vi "BuildFRF.vi"(8 "Method":enum16{"Sqrt(H1H2)", "H1", "H2"}(ring), 9 "Settings":T1={"Name of test"="ScratchPad", "Date"=timestamp(0 s since 1904-01-01), "Location"="Home", "Template"="ScratchPad", "Soundcard"="OCTA-CAPTURE", "resolution"=32, "Sampling rate"=48000, "Ch1 Gain "=25.0, "Ch2 Gain"=10.0, "Sample time (s)"=0.3, "Pre-trigger (s)"=0.001, "Hammer Threshold"=10.0, "Positions"=12, "Taps/Position"=5, "Set Names"="H,V", "Freq resolution"=1.0, "Hammer cutoff"=0.025, "Mic cutoff"=0.25, "Double bounce "=10.0, "Hammer Cal"=0.022, "dB Offset"=0.0, "Accel Cal"=10.0, "Vibrometer Cal"=1.0, "Mic Cal"=1.0, "Output"=2, "Voltage Cal"=1.0, "Vibrometer Port"="ASRL27::INSTR", "Range"=4, "High Pass"=2, "Bandwidth"=4, "X Range"=[], "Y Range"=[], "dB Spread"=0.0, "Trigger"=0, "Ch_1"=25, "Ch_2"=25, "flip?"=FALSE, "60Hz"=FALSE, "Time offset"=0.0, "Piezo Cal"=1.0, "Default Notes"=""} {"Ch_2" min=1 step=1; "Ch_1" min=1 max=100 step=1; "Trigger" items=["Hammer (force)", "Self-tap", "Spacebar"]; "Bandwidth" items=["1 kHz"=1, "5 kHz"=5, "10 kHz"=10, "25 kHz"=25, "50 kHz"=50, "100 kHz"=100]; "High Pass" items=["Off", "13 Hz", "104 Hz"]; "Range" items=["10 mm/s"=1, "20 mm/s"=2, "50 mm/s"=5, "100 mm/s"=10, "200 mm/s"=20, "500 mm/s"=50, "1 m/s"=100, "2 m/s"=200]; "Output" items=["Accelerometer", "Speed (from acceleration)", "Microphone", "Vibrometer", "Piezo"]; "Voltage Cal" format="%#_13g"; "Ch2 Gain" format="%#_13g"; "Ch1 Gain" format="%#_13g"; "Double bounce" min=0.0; "Mic cutoff" min=0.0 format="%#_4g"; "Hammer cutoff" min=0.0 format="%#_4g"; "Freq resolution" min=0.0; "Pre-trigger (s)" format="%#_13g"; "Date" format="%<%H:%M\n%d/%m/%y>T"; "resolution" items=["16 bit"=16, "24 bit"=24, "32 bit"=32]; "Sampling rate" items=["22050 samp/s"=22050, "44100 samp/s"=44100, "48000 samp/s"=48000]}, 10 "View":u16(ring) items=["Raw", "Volts", "Units (Pa, N, mm/s etc)"], 11 "Data In":waveform(dbl)[](array[waveform])=[{"t0"=timestamp(3613749982.386897 s since 1904-01-01), "dt"=2.0833333333333333e-05, "Y"=array[14400 elements]}, {"t0"=timestamp(3613749982.386897 s since 1904-01-01), "dt"=2.0833333333333333e-05, "Y"=array[14400 elements]}]) -> (0 "Average FRF":cluster{dbl, "df":dbl, dbl[]}[](graph)=[{1.0, "df"=1.0, array[24000 elements]}, {1.0, "df"=1.0, array[24000 elements]}], 1 "Microphone":cluster{dbl, "dt":dbl, "Y":dbl[]}[](graph)=[{0.0, "dt"=2.0833333333333333e-05, "Y"=array[14400 elements]}], 2 "Hammer":cluster{dbl, "dt":dbl, "Y":dbl[]}[](graph), 3 "Complex FRF":cluster{"t0":dbl, "dt":dbl, "Y":cdb[]}={"t0"=1.0, "dt"=1.0, "Y"=array[24000 elements]}, 4 "Microphone Spectra":cluster{"x0":dbl, "df":dbl, dbl[]}[](graph)=[{"x0"=1.0, "df"=1.0, array[24000 elements]}], 5 "Hammer Spectra":cluster{dbl, "df":dbl, "FFT {X}":dbl[]}[](graph)=[{1.0, "df"=1.0, "FFT {X}"=array[24000 elements]}])   [LabVIEW 2022 SP3]
uses:
  PreferencesControl.ctl
  Mic/Mic_Global.vi
panel:
  # "Always empty for TapTones because there is no hammer"
  # "Hz"
  # "dB"
  # "dB"
  # "sec"
  # "sec"
  # "mV/Pa"
  # "mV/m/s2"
  # "mV/mm/s"
  # "V/N"
  # "sec"
  # "sec"
  # "mV/N"
  # "a.u."
  # "a.u."
  # "sec"
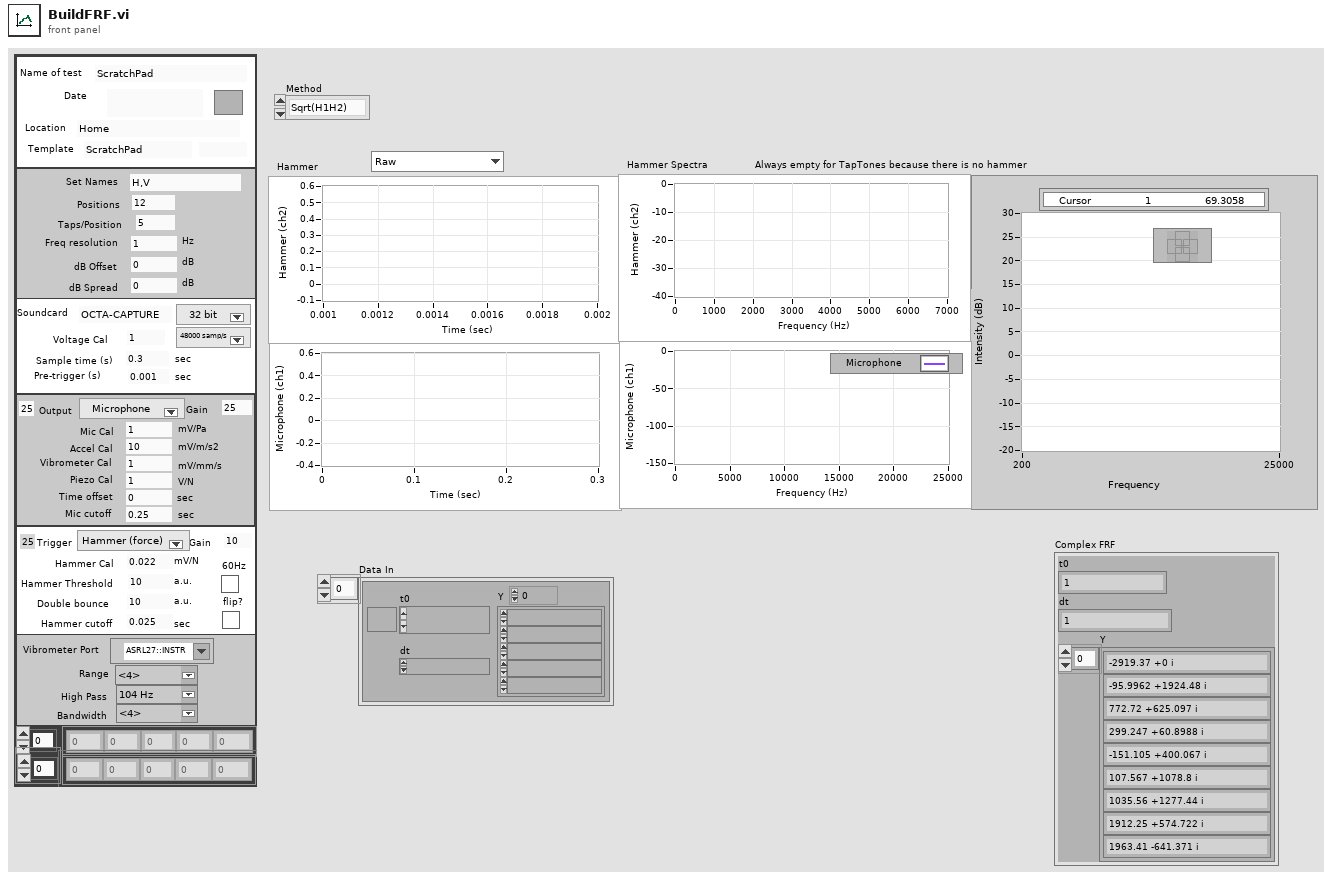
[diagram p1: front panel]
types:
  T1 = typedef "PreferencesControl.ctl" = cluster{"Name of test":string, "Date":timestamp, "Location":string, "Template":string, "Soundcard":string, "resolution":u16, "Sampling rate":u16, "Ch1 Gain ":dbl, "Ch2 Gain":dbl, "Sample time (s)":dbl, "Pre-trigger (s)":dbl, "Hammer Threshold":dbl, "Positions":i16, "Taps/Position":i16, "Set Names":string, "Freq resolution":dbl, "Hammer cutoff":dbl, "Mic cutoff":dbl, "Double bounce ":dbl, "Hammer Cal":dbl, "dB Offset":dbl, "Accel Cal":dbl, "Vibrometer Cal":dbl, "Mic Cal":dbl, "Output":u16, "Voltage Cal":dbl, "Vibrometer Port":refnum<visa-resource-name>, "Range":u16, "High Pass":u16, "Bandwidth":u16, "X Range":cluster{"Minimum":dbl, "Maximum":dbl, "Increment":dbl, "Minor Increment":dbl, "Start":dbl}[], "Y Range":cluster{"Minimum":dbl, "Maximum":dbl, "Increment":dbl, "Minor Increment":dbl, "Start":dbl}[], "dB Spread":dbl, "Trigger":u16, "Ch_1":u8, "Ch_2":u8, "flip?":bool, "60Hz":bool, "Time offset":dbl, "Piezo Cal":dbl, "Default Notes":string}
  T2 = cluster{"Alerts":bool, "Log X Axis":bool, "dB scale":bool, "Averaging":bool, "Fade":dbl, "Centroids?":bool}
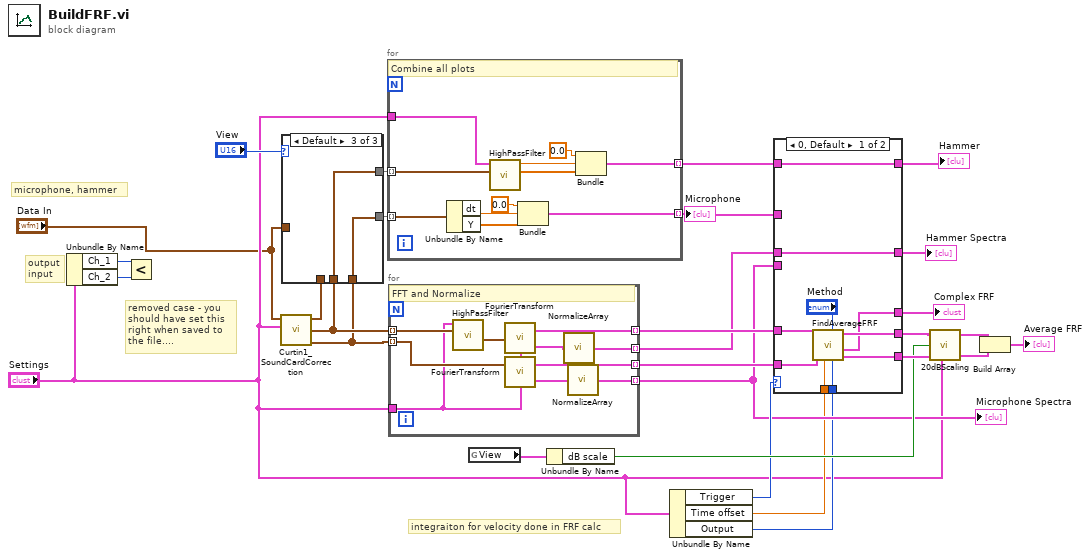
[diagram p0: block diagram]
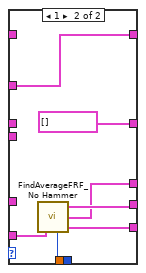
[diagram p2: hidden frame]
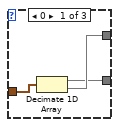
[diagram p3: hidden frame]
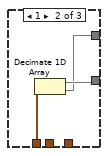
[diagram p4: hidden frame]
diagram:
  # "removed case - you \nshould have set this\nright when saved to \nthe file...."
  # "output\ninput"
  # "microphone, hammer"
  # "integraiton for velocity done in FRF calc"
  n1 = Unbundle By Name("Settings") -> ("Ch_1"=w3:u8, "Ch_2"=w2:u8)
  n2 = Less?(x=w3, y=w2) -> ()  [unwired: 1 out]
  n3 = call "Curtin1_SoundCardCorrection.vi"("Settings"="Settings", "Buffer in"="Data In") -> ("Microphone"=w14:waveform(dbl)[], "Hammer"=w15:waveform(dbl)[], "Volts Out"=w16:waveform(dbl)[])  [unwired: 4 in, 3 out]
  n4 = case shown="Default" "View" {
    tunnel: "Data In" -> [w32 _ _]
    tunnel: [w30 w34 w36] -> w18
    tunnel: [w31 w33 w37] -> w17
    tunnel: w16 -> [_ w35 _]
    tunnel: w15 -> [_ _ w37]
    tunnel: w14 -> [_ _ w36]
    frame 0 {
      n5 = Decimate 1D Array(w32) -> (w30:waveform(dbl)[], w31:waveform(dbl)[])
    }
    frame 1 {
      n6 = Decimate 1D Array(w35) -> (w34:waveform(dbl)[], w33:waveform(dbl)[])
    }
    frame Default {
    }
  }
  n7 = for {
    tunnel: [w46] -> w11 mode=indexing
    tunnel: w17 -> [w45] mode=indexing
    tunnel: w18 -> [w41] mode=indexing
    tunnel: [w40] -> w8 mode=indexing
    tunnel: "Settings" -> [w39]
    # "Combine all plots"
    n8 = Unbundle By Name(w41) -> ("dt"=w43:dbl, "Y"=w42:dbl[])
    n9 = call "HighPassFilter.vi"("Data"=w45, "Settings"=w39) -> ("Filtered X"=w38:dbl[], "dt"=w48:dbl)  [unwired: 7 in, 1 out]
    n10 = Bundle(0.0, "dt"=w43, "Y"=w42) -> (w40:cluster{dbl, "dt":dbl, "Y":dbl[]})  [unwired: 1 in]
    n11 = Bundle(0.0, "dt"=w48, "Filtered X"=w38) -> (w46:cluster{dbl, "dt":dbl, "Filtered X":dbl[]})  [unwired: 1 in]
  }
  "Microphone" <- w8
  n12 = for {
    tunnel: [w58] -> w27 mode=indexing
    tunnel: [w57] -> w28 mode=indexing
    tunnel: [w53] -> w12 mode=indexing
    tunnel: [w55] -> w7 mode=indexing
    tunnel: w15 -> [w51] mode=indexing
    tunnel: w14 -> [w52] mode=indexing
    tunnel: "Settings" -> [w50]
    # "FFT and Normalize"
    n13 = call "HighPassFilter.vi"("Data"=w51, "Settings"=w50) -> ("Data out"=w49:waveform(dbl))  [unwired: 7 in, 2 out]
    n14 = call "FourierTransform.vi"("Settings"=w50, "Data"=w49) -> ("Magnitude of Spectrum"=w54:cluster{"x0":dbl, "df":dbl, dbl[]}, "FFT"=w58:cluster{dbl, "df":dbl, "FFT {X}":cdb[]})  [unwired: 2 in]
    n15 = call "FourierTransform.vi"("Settings"=w50, "Data"=w52) -> ("Magnitude of Spectrum"=w56:cluster{"x0":dbl, "df":dbl, dbl[]}, "FFT"=w57:cluster{dbl, "df":dbl, "FFT {X}":cdb[]})  [unwired: 2 in]
    n16 = call "NormalizeArray.vi"("Magnitude of Spectrun"=w54) -> ("Magnitude of Spectrun"=w53:cluster{"x0":dbl, "df":dbl, dbl[]})
    n17 = call "NormalizeArray.vi"("Magnitude of Spectrun"=w56) -> ("Magnitude of Spectrun"=w55:cluster{"x0":dbl, "df":dbl, dbl[]})
  }
  "Microphone Spectra" <- w7
  n18 = global read "Mic_Global.vi" "View"() -> (w21:T2)
  n19 = Unbundle By Name(w21) -> ("dB scale"=w20:bool)
  n20 = Unbundle By Name("Settings") -> ("Trigger"=w13:u16, "Time offset"=w5:dbl, "Output"=w6:u16)
  n21 = case shown="0, Default" w13 {
    tunnel: w28 -> [w60 w75]
    tunnel: w27 -> [w68 _]
    tunnel: [w67 w74] -> w26
    tunnel: [w64 w73] -> w25
    tunnel: [w62 w70] -> w22
    tunnel: w12 -> [w65 _]
    tunnel: w11 -> [w66 _]
    tunnel: [w66 w72] -> w10
    tunnel: [w65 cluster{dbl, "dt":dbl, "Y":dbl[]}[] []] -> w9
    tunnel: w8 -> [_ w72]
    tunnel: w7 -> [_ _]
    tunnel: w6 -> [w63 w69]
    tunnel: w5 -> [w59 _]
    frame 0, Default {
      n22 = call "FindAverageFRF.vi"("Output"=w63, "Method"="Method", "delay"=w59, "Microphone Spectrum"=w60, "Hammer Spectrum"=w68) -> ("Coherence"=w67:cluster{"x0":dbl, "df":dbl, dbl[]}, "Complex FRF"=w62:cluster{"t0":dbl, "dt":dbl, "Y":cdb[]}, "Average FRF"=w64:cluster{"x0":dbl, "df":dbl, dbl[]})  [unwired: 4 in]
    }
    frame 1 {
      n23 = call "FindAverageFRF_No Hammer.vi"("Output"=w69, "Microphone Spectrum"=w75) -> ("Coherence"=w74:cluster{"x0":dbl, "df":dbl, dbl[]}, "Complex FRF"=w70:cluster{"t0":dbl, "dt":dbl, "Y":cdb[]}, "Average FRF"=w73:cluster{"x0":dbl, "df":dbl, dbl[]})  [unwired: 2 in]
    }
  }
  "Hammer Spectra" <- w9
  "Hammer" <- w10
  "Complex FRF" <- w22
  n24 = call "20dBScaling.vi"("Average FRF in"=w25, "dB?"=w20, "Coherence in"=w26, "Settings"="Settings") -> ("Average FRF out"=w24:cluster{"x0":dbl, "df":dbl, dbl[]}, "Coherence out"=w23:cluster{"x0":dbl, "df":dbl, dbl[]})  [unwired: 2 in]
  n25 = Build Array(w24, w23) -> (→"Average FRF":cluster{"x0":dbl, "df":dbl, dbl[]}[])
